vi "LoadWaveform.vi"(5 "offset":dbl format="%0.2p", 6 "phase":dbl format="%.2p", 7 "signal type":T1(ring), 8 "frequency":dbl=10.0 format="%0.2p", 9 "amplitude":dbl=1.0 format="%0.2p", 10 "Channel":i32, 11 "Handle":u32) -> (3 "FT_Status":u32(ring) items=["FT_OK", "FT_INVALID_HANDLE", "FT_DEVICE_NOT_FOUND", "FT_DEVICE_NOT_OPENED", "FT_IO_ERROR", "FT_INSUFFICIENT_RESOURCES", "FT_INVALID_PARAMETER", "FT_INVALID_BAUD_RATE", "FT_DEVICE_NOT_OPENED_FOR_ERASE", "FT_DEVICE_NOT_OPENED_FOR_WRITE", "FT_FAILED_TO_WRITE_DEVICE", "FT_EEPROM_READ_FAILED", "FT_EEPROM_WRITE_FAILED", "FT_EEPROM_ERASE_FAILED", "FT_EEPROM_NOT_PRESENT", "FT_EEPROM_NOT_PROGRAMMED", "FT_INVALID_ARGS", "FT_NOT_SUPPORTED", "FT_OTHER_ERROR"])   [LabVIEW 2017]
uses:
  <vilib>/measure/NI_MABase.lvlib
panel:
  in  "sampling info":cluster{"Fs":dbl, "#s":dbl}={"Fs"=1000.0, "#s"=1000.0} {"Fs" format="%.2p"}
  out "Bytes Written":u32
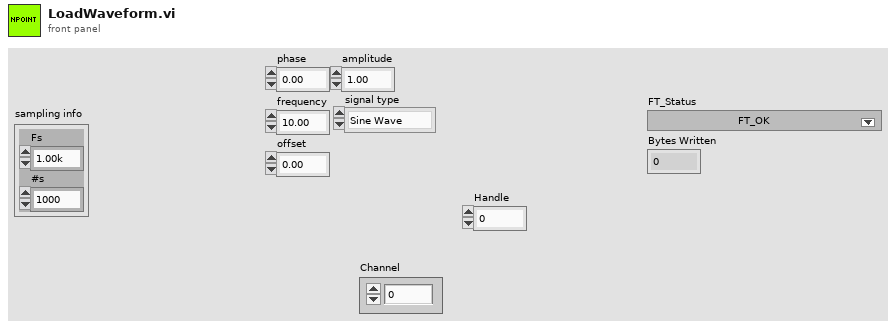
[diagram p1: front panel]
types:
  T1 = enum16{"Sine Wave", "Triangle Wave", "Square Wave", "Sawtooth Wave"}
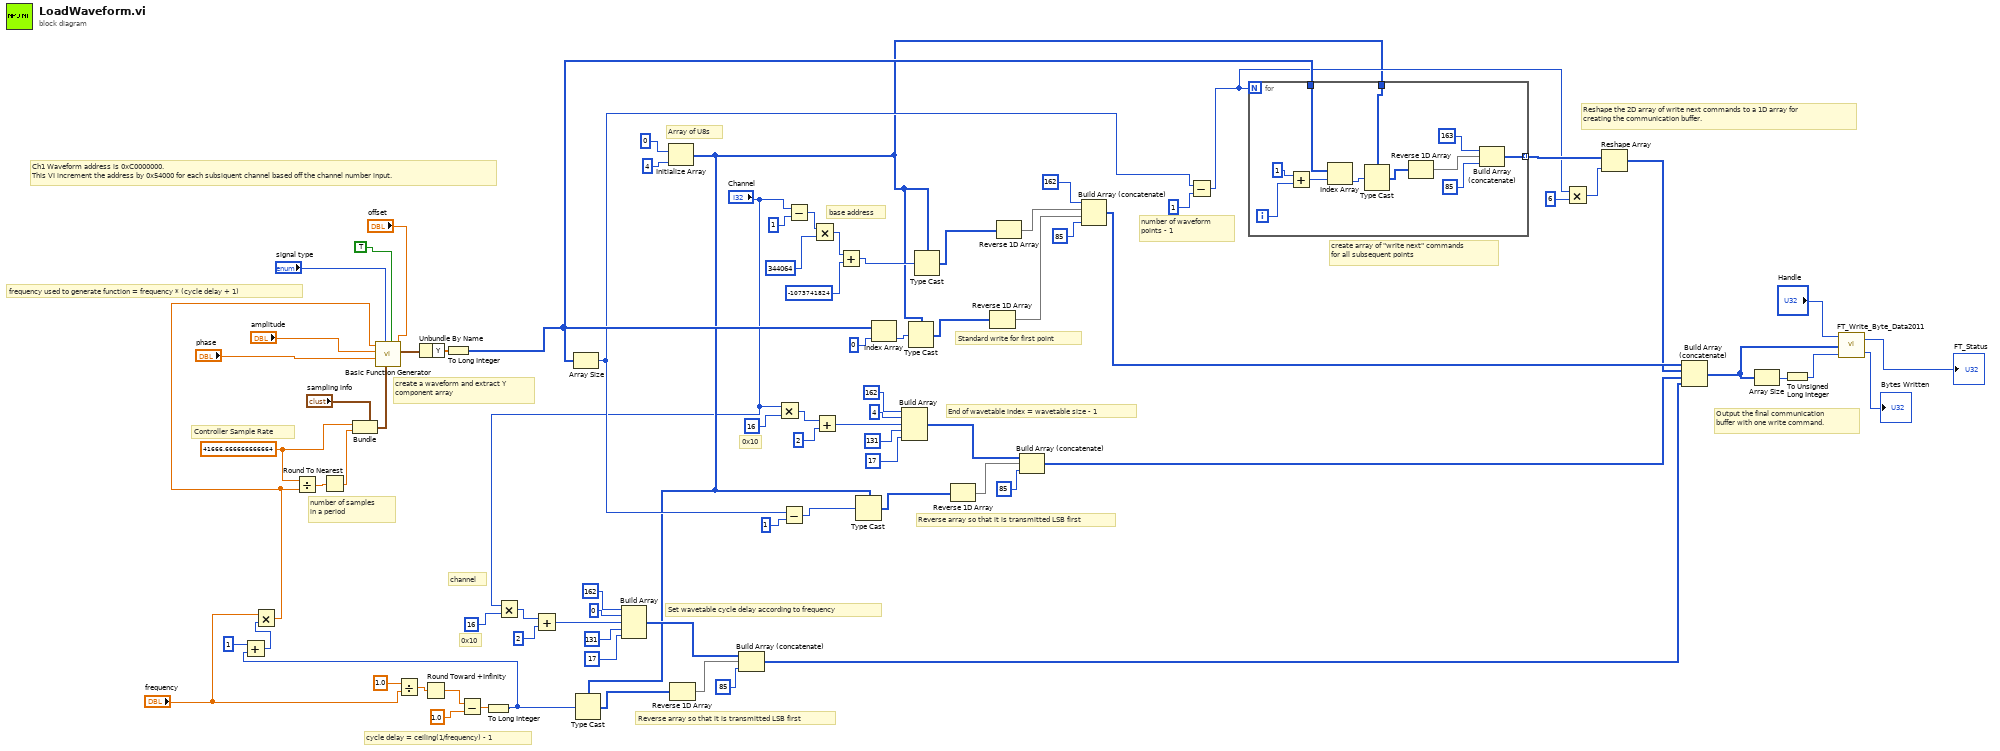
[diagram p0: block diagram]
diagram:
  w71 = 41666.666666666664 ("Fs")
  # "frequency used to generate function = frequency * (cycle delay + 1)"
  # "cycle delay = ceiling(1/frequency) - 1"
  # "channel"
  # "Set wavetable cycle delay according to frequency"
  # "Reverse array so that it is transmitted LSB first"
  # "0x10"
  # "Output the final communication\nbuffer with one write command."
  # "Reshape the 2D array of write next commands to a 1D array for \ncreating the communication buffer."
  # "Standard write for first point"
  # "create array of \"write next\" commands\nfor all subsequent points"
  # "End of wavetable index = wavetable size - 1"
  # "Reverse array so that it is transmitted LSB first"
  # "0x10"
  # "Array of U8s"
  # "number of waveform\npoints - 1"
  # "base address"
  # "create a waveform and extract Y\ncomponent array"
  # "number of samples\nin a period"
  # "Controller Sample Rate"
  # "Ch1 Waveform address is 0xC0000000.\nThis VI increment the address by 0x54000 for each subsiquent channel based off the channel number input."
  n1 = Divide(x=1.0, y="frequency") -> (x/y=w3:dbl)
  n2 = Round Toward +Infinity(x=w3) -> (ceil(x): smallest int >= x=w2:dbl)
  n3 = Subtract(x=w2, y=1.0) -> (x-y=w4:dbl)
  n4 = To Long Integer(number=w4) -> (32bit integer=w8:i32)
  n5 = Add(x=1, y=w8) -> (x+y=w9:i32)
  n6 = Multiply(x="frequency", y=w9) -> (x*y=w6:dbl)
  n7 = Divide(x=w71, y=w6) -> (x/y=w75:dbl)
  n8 = Round To Nearest(number=w75) -> (nearest integer value=w74:dbl)
  n9 = Bundle(cluster="sampling info", "Fs"=w71, "#s"=w74) -> (w76:cluster{"Fs":dbl, "#s":dbl})
  n10 = call <vilib>:"Basic Function Generator.vi"("offset"="offset", "reset signal"=TRUE, "sampling info"=w76, "signal type"="signal type", "phase"="phase", "amplitude"="amplitude", "frequency"=w6) -> ("signal out"=w78:waveform(dbl))  [unwired: 2 in, 2 out]
  n11 = Unbundle By Name ("Get Waveform Components")(w78) -> ("Y"=w73:dbl[])
  n12 = To Long Integer(number=w73) -> (32bit integer=w49:i32[])
  n13 = Multiply(x="Channel", y=u8 16) -> (x*y=w24:i32)
  n14 = Add(x=w24, y=u8 2 ("element")) -> (x+y=w25:i32)
  n15 = Array Size(array=w49) -> (size(s)=w28:i32)
  n16 = Build Array(u8 162 ("element"), u8 0 ("element"), w25, u8 131 ("element"), u8 17 ("element")) -> (w18:i32[])
  n17 = Initialize Array(u8 0, 4 ("dimension size")) -> (w11:u8[])
  n18 = Type Cast(type=w11, x=w8) -> (*(type *) &x=w20:u8[])
  n19 = Reverse 1D Array(array=w20) -> (reversed array=w21:u8[])
  n20 = Build Array (concatenate)(w18, w21, u8 85 ("element")) -> (w1:i32[])
  n21 = Multiply(x="Channel", y=u8 16) -> (x*y=w31:i32)
  n22 = Subtract(x=w28, y=1) -> (x-y=w26:i32)
  n23 = Subtract(x="Channel", y=1) -> (x-y=w64:i32)
  n24 = Multiply(x=w64, y=344064) -> (x*y=w63:i32)
  n25 = Add(x=w31, y=u8 2 ("element")) -> (x+y=w30:i32)
  n26 = Add(x=w63, y=-1073741824) -> (x+y=w51:i32)
  n27 = Type Cast(type=w11, x=w26) -> (*(type *) &x=w35:u8[])
  n28 = Index Array(array=w49, index=0) -> (element=w61:i32)
  n29 = Build Array(u8 162 ("element"), u8 4 ("element"), w30, u8 131 ("element"), u8 17 ("element")) -> (w37:i32[])
  n30 = Type Cast(type=w11, x=w61) -> (*(type *) &x=w57:u8[])
  n31 = Type Cast(type=w11, x=w51) -> (*(type *) &x=w55:u8[])
  n32 = Reverse 1D Array(array=w35) -> (reversed array=w34:u8[])
  n33 = Reverse 1D Array(array=w57) -> (reversed array=w58:u8[])
  n34 = Reverse 1D Array(array=w55) -> (reversed array=w56:u8[])
  n35 = Build Array (concatenate)(w37, w34, u8 85 ("element")) -> (w29:i32[])
  n36 = Build Array (concatenate)(u8 162 ("element"), w56, w58, u8 85 ("element")) -> (w47:u8[])
  n37 = Subtract(x=w28, y=1) -> (x-y=w45:i32)
  n38 = for {
    N: w45 -> [_]
    tunnel: w11 -> [w91]
    tunnel: w49 -> [w90]
    tunnel: [w84] -> w46 mode=indexing
    i -> [w85]
    n39 = Add(x=1 ("y"), y=w85) -> (x+y=w89:i32)
    n40 = Index Array(array=w90, index=w89) -> (element=w93:i32)
    n41 = Type Cast(type=w91, x=w93) -> (*(type *) &x=w92:u8[])
    n42 = Reverse 1D Array(array=w92) -> (reversed array=w88:u8[])
    n43 = Build Array (concatenate)(u8 163 ("element"), w88, u8 85 ("element")) -> (w84:u8[])
  }
  n44 = Multiply(x=w45, y=6) -> (x*y=w43:i32)
  n45 = Reshape Array "Reshape Array"(w46, w43) -> (w42:u8[])
  n46 = Build Array (concatenate)(w47, w42, w29, w1) -> (w48:i32[])
  n47 = Array Size(array=w48) -> (size(s)=w83:i32)
  n48 = To Unsigned Long Integer(number=w83) -> (unsigned 32bit integer=w81:u32)
  n49 = call "FT_Write_Byte_Data2011.vi"("Bytes To Write"=w81, "Buffer"=w48, "Handle"="Handle") -> ("Bytes Written"=→"Bytes Written":u32, "FT_Status"=→"FT_Status":u32)
